vi "Test Extract ARGB.vi"(8 "error in (no error)":errorcluster) -> (0 "error out":errorcluster, 3 "Test Case Out":refnum<class "Image.lvclass">)   [LabVIEW 2020, in "g_ar_toolkit.test.lvlib" / "Image.lvclass"]
uses:
  Image.lvclass
  C:/Program Files (x86)/National Instruments/LabVIEW 2020/vi.lib/Astemes/LUnit/Test Case.lvclass
  g_ar_toolkit.common/Image Size (Integer).ctl
  <vilib>/Astemes/LUnit/Test Case.lvclass/Test Case.ctl
  g_ar_toolkit.image/New Image (Greyscale).vi
  g_ar_toolkit.image/Get Channel (Red).vi
  g_ar_toolkit.image/Get Channel (Alpha).vi
  g_ar_toolkit.image/Get Channel (Green).vi
  g_ar_toolkit.image/Get Channel (Blue).vi
  4993e8ee-a06a-463a-9684-69129f64d5ce.vi
  g_ar_toolkit.image/New Image (ARGB).vi
  g_ar_toolkit.image/Copy Array to Image.vi
  g_ar_toolkit.image/Copy Array to Image (ARGB).vi
  g_ar_toolkit.image/New Image (Greyscale).vi/6598b9e0-8a08-46f5-91fd-ca1b87217137.vi
  g_ar_toolkit.image/ARGBExtractChannel.vi
  <vilib>/Astemes/LUnit/Append Pass Result.vi
  <vilib>/Astemes/LUnit/Append Fail Result.vi
  <vilib>/Astemes/LUnit/Describe Comparison.vi
  4993e8ee-a06a-463a-9684-69129f64d5ce.vi/9c5d11cd-9439-4240-a1ee-d9baace9c924.vi
  g_ar_toolkit.image/New Image (ARGB).vi/3321fa97-f432-4e1e-8db9-a0df79aed21b.vi
  g_ar_toolkit.image/ARGB Colour to U32 Pixel Value.vi
  <vilib>/Astemes/LUnit/Run In UI.vi
  <vilib>/Utility/error.llb/Clear Errors.vi
  g_ar_toolkit.common/Module Path.vi
  <vilib>/Utility/error.llb/Error Cluster From Error Code.vi
  <vilib>/picture/pixmap.llb/Flatten Pixmap.vi
  <vilib>/Astemes/LUnit/Describe Variant.vi
  Image.lvclass/Image.ctl
  g_ar_toolkit.image/g_ar_toolkit.image.lvlib
  g_ar_toolkit.common/g_ar_toolkit.common.lvlib
panel:
  in  "Test Case in":refnum<class "Image.lvclass">
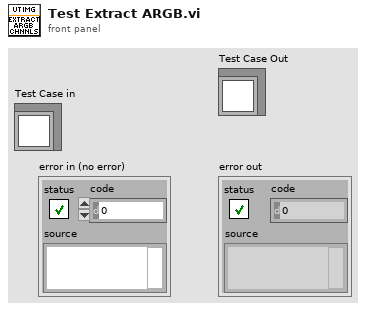
[diagram p1: front panel]
types:
  T1 = typedef "g_ar_toolkit.common.lvlib/Image Size (Integer).ctl" = cluster{"Width":u16, "Height":u16}
  T2 = typedef "g_ar_toolkit.image.lvlib/ARGB Image.ctl" = refnum<data-value>
  T3 = typedef "g_ar_toolkit.image.lvlib/Greyscale Image.ctl" = refnum<data-value>
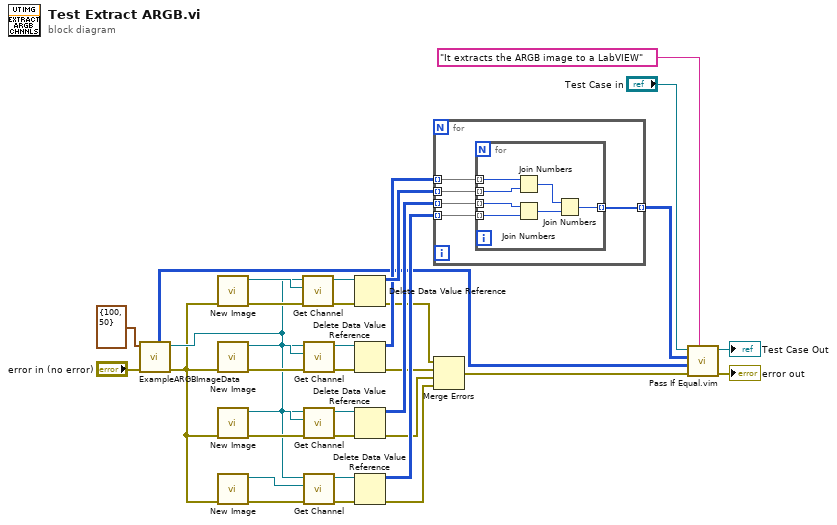
[diagram p0: block diagram]
diagram:
  n1 = call "ExampleARGBImageData.vi"("error in (no error)"="error in (no error)", "Image Size"=T1 {"Width"=100, "Height"=50} ("Preallocated Image Size (Default - 0,0)")) -> ("error out"=w2:errorcluster, "Data Value Reference out"=w3:T2, "ARGB Array Data"=w1:u32[][])  [unwired: 6 in, 1 out]
  n2 = call-poly "New Image.vi"("error in (no error)"=w2) -> ("error out"=w20:errorcluster, "New Greyscale Image"=w33:T3)  [unwired: 9 in]
  n3 = call-poly "New Image.vi"("error in (no error)"=w2) -> ("error out"=w14:errorcluster, "New Greyscale Image"=w30:T3)  [unwired: 9 in]
  n4 = call-poly "New Image.vi"("error in (no error)"=w2) -> ("error out"=w12:errorcluster, "New Greyscale Image"=w32:T3)  [unwired: 9 in]
  n5 = call-poly "New Image.vi"("error in (no error)"=w2) -> ("error out"=w17:errorcluster, "New Greyscale Image"=w31:T3)  [unwired: 9 in]
  n6 = call-poly "Get Channel.vi"("error in (no error)"=w20, "Greyscale Image Destination"=w33, "ARGB Image Source"=w3) -> ("error out"=w19:errorcluster, "Greyscale Image Destination (Duplicate)"=w29:T3)  [unwired: 7 in]
  n7 = call-poly "Get Channel.vi"("error in (no error)"=w14, "Greyscale Image Destination"=w30, "ARGB Image Source"=w3) -> ("error out"=w13:errorcluster, "Greyscale Image Destination (Duplicate)"=w26:T3)  [unwired: 7 in]
  n8 = call-poly "Get Channel.vi"("error in (no error)"=w12, "Greyscale Image Destination"=w32, "ARGB Image Source"=w3) -> ("error out"=w11:errorcluster, "Greyscale Image Destination (Duplicate)"=w28:T3)  [unwired: 7 in]
  n9 = call-poly "Get Channel.vi"("error in (no error)"=w17, "Greyscale Image Destination"=w31, "ARGB Image Source"=w3) -> ("error out"=w10:errorcluster, "Greyscale Image Destination (Duplicate)"=w27:T3)  [unwired: 7 in]
  n10 = Delete Data Value Reference(data value reference=w29, error in=w19) -> (data value=w25:u8[][], error out=w18:errorcluster)
  n11 = Delete Data Value Reference(data value reference=w26, error in=w13) -> (data value=w22:u8[][], error out=w9:errorcluster)
  n12 = Delete Data Value Reference(data value reference=w28, error in=w11) -> (data value=w24:u8[][], error out=w8:errorcluster)
  n13 = Delete Data Value Reference(data value reference=w27, error in=w10) -> (data value=w23:u8[][], error out=w7:errorcluster)
  n14 = for {
    tunnel: w25 -> [w40] mode=indexing
    tunnel: w24 -> [w39] mode=indexing
    tunnel: w23 -> [w38] mode=indexing
    tunnel: w22 -> [w37] mode=indexing
    tunnel: [w36] -> w21 mode=indexing
    n15 = for {
      tunnel: w40 -> [w46] mode=indexing
      tunnel: w39 -> [w45] mode=indexing
      tunnel: w38 -> [w44] mode=indexing
      tunnel: w37 -> [w47] mode=indexing
      tunnel: [w41] -> w36 mode=indexing
      n16 = Join Numbers(hi=w47, lo=w46) -> ((hi.lo)=w43:u16)
      n17 = Join Numbers(hi=w45, lo=w44) -> ((hi.lo)=w42:u16)
      n18 = Join Numbers(hi=w43, lo=w42) -> ((hi.lo)=w41:u32)
    }
  }
  n19 = Merge Errors(w18, w9, w8, w7) -> (w6:errorcluster)
  n20 = call "Pass If Equal.vim"("Description"="It extracts the ARGB image to a LabVIEW", "error in (no error)"=w6, "Actual"=w1, "Expected"=w21, "LUnit Test Case In"="Test Case in") -> ("error out"=→"error out":errorcluster, "LUnit Test Case Out"=→"Test Case Out":refnum<class "Image.lvclass">)  [unwired: 5 in]
